vi "UDP 쓰기.vi"() -> ()   [LabVIEW 2014]
panel:
  in  "정지":bool
  in  "이름":string="121.139.99.186"
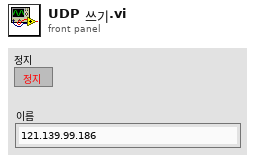
[diagram p1: front panel]
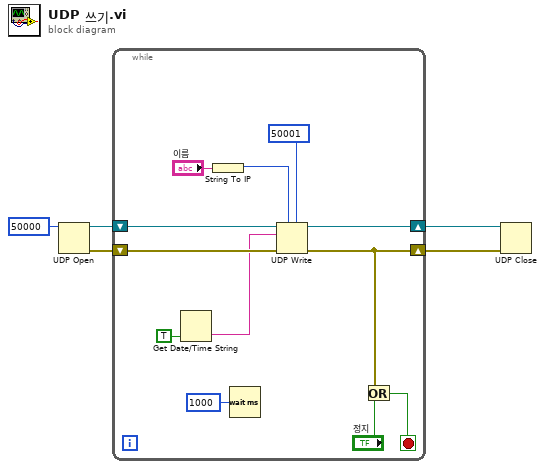
[diagram p0: block diagram]
diagram:
  n1 = UDP Open(11:u16 50000 ("포트")) -> (port=w5:refnum<k16>, 0:w3:errorcluster)  [unwired: 4 in, 1 out]
  n2 = while {
    shift-right: [w16] -> w4
    shift-left: w5 -> [w17]
    shift-right: [w7] -> w2
    shift-left: w3 -> [w15]
    stop <- w9 stop-if-true
    n3 = Get Date/Time String(want seconds? (F)=TRUE ("초 보이기? (거짓)")) -> (time string=w12:string)  [unwired: 2 in, 1 out]
    n4 = String To IP(1:"이름") -> (0:w10:u32)
    n5 = Wait (ms)(milliseconds to wait=u32 1000 ("대기 시간(ms)")) -> ()  [unwired: 1 out]
    n6 = UDP Write(address=w10, port or service name=u16 50001 ("포트 또는 서비스 이름"), connection ID=w17, data in=w12, 8:w15) -> (error out=w7:errorcluster, 3:w16:refnum<k16>)  [unwired: 1 in]
    n7 = Or(x=w7, y="정지") -> (x .or. y?=w9:bool)
  }
  n8 = UDP Close(connection ID=w4, 8:w2) -> ()  [unwired: 2 out]
